vi "CTR_DataStream_Init.vi"(0 "CTR Endpoint":string="CTR001", 5 "DAQ Endpoint":string, 7 "CTR IP Addr":string, 9 "DAQ IP Addr":string, 11 "error in":errorcluster, 12 "timeout ms":i32=-1, 13 "Buffer":i32) -> (4 "writer endpoint":refnum<k21>, 6 "reader endpoint":refnum<k21>, 15 "error out":errorcluster)   [LabVIEW 2024]
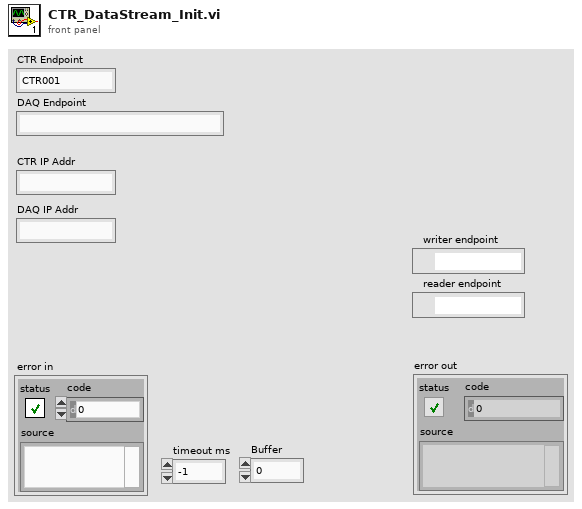
[diagram p1: front panel]
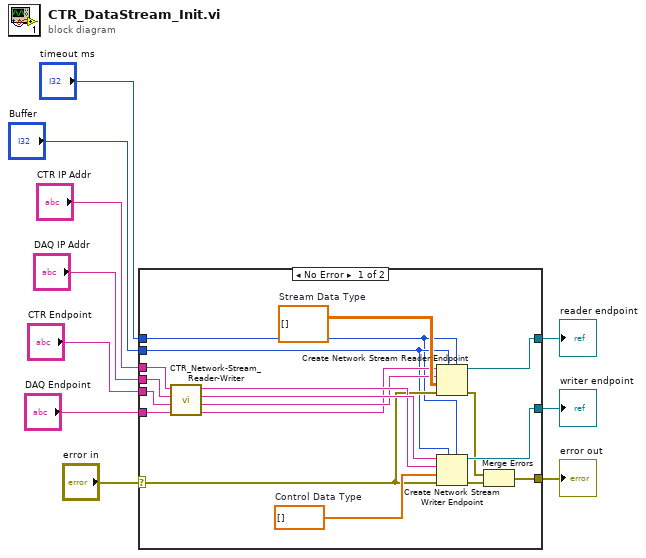
[diagram p0: block diagram]
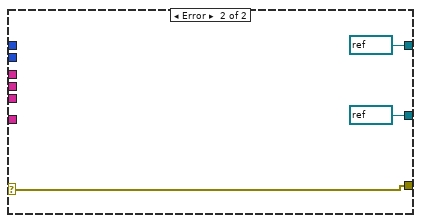
[diagram p2: hidden frame]
diagram:
  n1 = case shown="No Error" "error in" {
    selector: "error in" -> [w18 w29]
    tunnel: [w17 w29] -> w10
    tunnel: "CTR Endpoint" -> [w23 _]
    tunnel: "DAQ Endpoint" -> [w26 _]
    tunnel: "Buffer" -> [w12 _]
    tunnel: [w27 refnum<k21> refnum ("writer endpoint")] -> w6
    tunnel: [w20 refnum<k21> refnum ("reader endpoint")] -> w2
    tunnel: "DAQ IP Addr" -> [w24 _]
    tunnel: "CTR IP Addr" -> [w25 _]
    tunnel: "timeout ms" -> [w11 _]
    frame No Error {
      w19 = dbl[][] []  # Stream Data Type
      w28 = dbl[] []  # Control Data Type
      n2 = call "CTR_Network-Stream_Reader-Writer.vi"("DAQ Endpoint"=w26, "CTR Endpoint"=w23, "DAQ IP Addr"=w24, "CTR IP Addr"=w25) -> ("//CTR IP Addr:CTR000/DAQ000-Data"=w13:string, "//DAQ IP Addr:DAQ000/DAQ000-Data"=w14:string, "//CTR IP Addr:CTR000/DAQ000-Control"=w22:string, "//DAQ IP Addr:DAQ000/DAQ000-Control"=w21:string)  [unwired: 4 in]
      n3 = Create Network Stream Reader Endpoint(5:w11, 7:w12, 8:w18, 9:w19, 10:w14, 11:w13) -> (0:w15:errorcluster, 3:w20:refnum<k21>)  [unwired: 1 in]
      n4 = Create Network Stream Writer Endpoint(5:w11, 7:w12, 8:w18, 9:w28, 10:w21, 11:w22) -> (0:w16:errorcluster, 3:w27:refnum<k21>)  [unwired: 1 in]
      n5 = Merge Errors(w15, w16) -> (w17:errorcluster)
    }
    frame Error {
    }
  }
  "error out" <- w10
  "writer endpoint" <- w6
  "reader endpoint" <- w2
